vi "Handle Web service.vi"(7 "Server Name":string="3 phase testbench", 11 "Web Request in":refnum<class "Web Request.lvclass">) -> ()   [LabVIEW 2025, in "MCP Server.lvlib"]
doc: "Use this VI in your LabVIEW Webservice inside a POST Method of any name. Just connect the Web Service reference, and the mcp server toolkit will handle all requests coming in through this method."
uses:
  MCP Server.lvlib
  <vilib>/wsapi/Web Request.lvclass
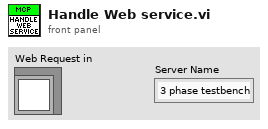
[diagram p1: front panel]
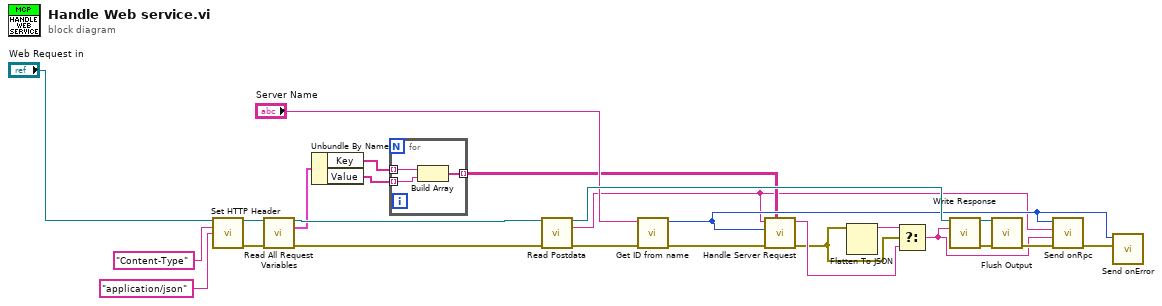
[diagram p0: block diagram]
diagram:
  n1 = call <vilib>:"Set HTTP Header.vi"("LabVIEW Web Service Request"="Web Request in", "header"="Content-Type", "header value"="application/json") -> ("LabVIEW Web Service Request out"=w5:refnum<class "Web Request.lvclass">, "error out"=w8:errorcluster)  [unwired: 11 in]
  n2 = call <vilib>:"Read All Request Variables.vi"("LabVIEW Web Service Request"=w5, "error in (no error)"=w8) -> ("LabVIEW Web Service Request out"=w12:refnum<class "Web Request.lvclass">, "request variables"=w4:cluster{"Key":string[], "Value":string[]}, "error out"=w13:errorcluster)  [unwired: 11 in]
  n3 = Unbundle By Name(w4) -> ("Key"=w3:string[], "Value"=w2:string[])
  n4 = for {
    tunnel: [w28] -> w11 mode=indexing
    tunnel: w3 -> [w27] mode=indexing
    tunnel: w2 -> [w26] mode=indexing
    n5 = Build Array(w27, w26) -> (w28:string[])
  }
  n6 = call <vilib>:"Read Postdata.vi"("LabVIEW Web Service Request"=w12, "error in (no error)"=w13) -> ("LabVIEW Web Service Request out"=w24:refnum<class "Web Request.lvclass">, "postdata"=w1:string, "error out"=w15:errorcluster)  [unwired: 11 in]
  n7 = call "Get ID from name.vi"("error in (no error)"=w15, "Name"="Server Name") -> ("error out"=w16:errorcluster, "id out"=w22:i32)  [unwired: 7 in, 1 out]
  n8 = call "Handle Server Request.vi"("parameters"=w11, "error in (no error)"=w16, "id in"=w22, "request"=w1) -> ("error out"=w10:errorcluster, "response"=w17:string)  [unwired: 6 in]
  n9 = Flatten To JSON(anything=w10) -> (JSON string=w9:string)  [unwired: 2 in, 1 out]
  n10 = Select(t=w9, s=w10, f=w17) -> (s? t:f=w18:string)
  n11 = call <vilib>:"Write Response.vi"("LabVIEW Web Service Request"=w24, "response string"=w18) -> ("LabVIEW Web Service Request out"=w19:refnum<class "Web Request.lvclass">, "error out"=w20:errorcluster)  [unwired: 12 in]
  n12 = call <vilib>:"Flush Output.vi"("LabVIEW Web Service Request"=w19, "error in (no error)"=w20) -> ("error out"=w21:errorcluster)  [unwired: 12 in, 1 out]
  n13 = call "Send onRpc.vi"("error in (no error)"=w21, "response"=w18, "request"=w1, "id"=w22) -> ("error out"=w23:errorcluster)  [unwired: 7 in]
  n14 = call "Send onError.vi"("error to report"=w23, "id"=w22) -> ()  [unwired: 9 in, 1 out]
